vi "niRFUtil WFM Bit Correlator.vi"(3 "Samples (-1 = All)":i32=-1, 4 "Bit Mask":T1 min=0, 5 "Bit Stream In":T1 min=0) -> (1 "Sync Index":u32, 2 "Bit Stream Out":T1 min=0)   [LabVIEW 2015, in "niRFUtil.lvlib"]
doc: "(c) Copyright 2006, National Instruments, Inc. This VI may not be duplicated, sold, or distributed without written consent from National Instruments."
uses:
  niRFUtil.lvlib
  Includes/niRFUtil INC Bit Array.ctl
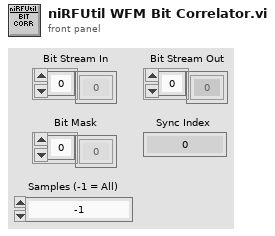
[diagram p1: front panel]
types:
  T1 = typedef "niRFUtil.lvlib/niRFUtil INC Bit Array.ctl" = i8[]
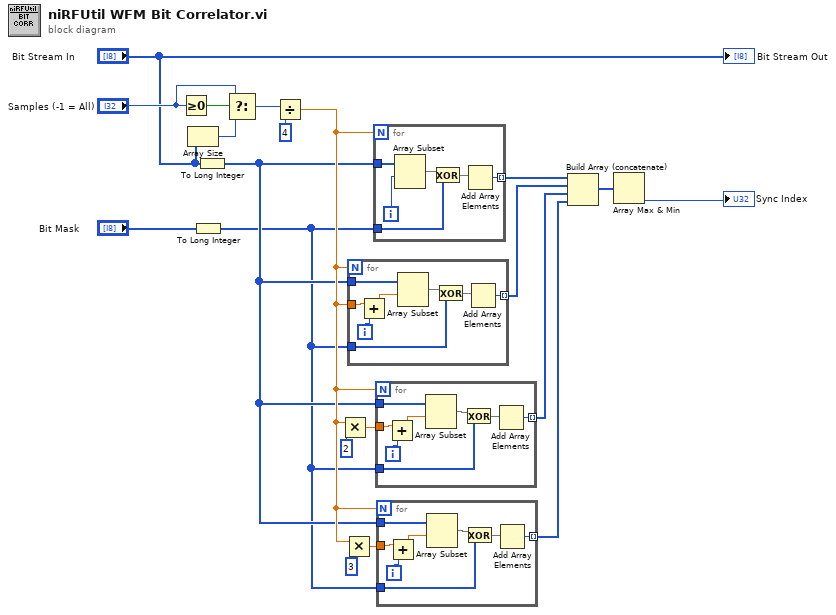
[diagram p0: block diagram]
diagram:
  n1 = Greater Or Equal To 0?(x="Samples (-1 = All)") -> (x >= 0?=w10:bool)
  n2 = Array Size(array="Bit Stream In") -> (size(s)=w9:i32)
  n3 = To Long Integer(number="Bit Mask") -> (32bit integer=w1:i32[])
  n4 = To Long Integer(number="Bit Stream In") -> (32bit integer=w2:i32[])
  n5 = Select(t="Samples (-1 = All)", s=w10, f=w9) -> (s? t:f=w8:i32)
  n6 = Divide(x=w8, y=4 ("x")) -> (x/y=w12:dbl)
  n7 = Multiply(x=w12, y=2) -> (x*y=w18:dbl)
  n8 = Multiply(x=w12, y=3) -> (x*y=w16:dbl)
  n9 = for {
    N: w12 -> [_]
    tunnel: w2 -> [w26]
    tunnel: w1 -> [w23]
    tunnel: [w27] -> w19 mode=indexing
    tunnel: w12 -> [w21]
    i -> [w24]
    n10 = Add(x=w21, y=w24) -> (x+y=w22:dbl)
    n11 = Array Subset(array=w26, index=w22) -> (w25:i32[])  [unwired: 1 in]
    n12 = Exclusive Or(1:w23, 2:w25) -> (0:w28:i32[])
    n13 = Add Array Elements(numeric array=w28) -> (sum=w27:i32)
  }
  n14 = for {
    N: w12 -> [_]
    tunnel: w2 -> [w32]
    tunnel: w1 -> [w29]
    tunnel: [w33] -> w20 mode=indexing
    i -> [w30]
    n15 = Array Subset(array=w32, index=w30) -> (w31:i32[])  [unwired: 1 in]
    n16 = Exclusive Or(1:w29, 2:w31) -> (0:w34:i32[])
    n17 = Add Array Elements(numeric array=w34) -> (sum=w33:i32)
  }
  n18 = for {
    N: w12 -> [_]
    tunnel: w2 -> [w40]
    tunnel: w1 -> [w37]
    tunnel: [w41] -> w14 mode=indexing
    tunnel: w18 -> [w35]
    i -> [w38]
    n19 = Add(x=w35, y=w38) -> (x+y=w36:dbl)
    n20 = Array Subset(array=w40, index=w36) -> (w39:i32[])  [unwired: 1 in]
    n21 = Exclusive Or(1:w37, 2:w39) -> (0:w42:i32[])
    n22 = Add Array Elements(numeric array=w42) -> (sum=w41:i32)
  }
  n23 = for {
    N: w12 -> [_]
    tunnel: w2 -> [w48]
    tunnel: w1 -> [w45]
    tunnel: [w49] -> w13 mode=indexing
    tunnel: w16 -> [w43]
    i -> [w46]
    n24 = Add(x=w43, y=w46) -> (x+y=w44:dbl)
    n25 = Array Subset(array=w48, index=w44) -> (w47:i32[])  [unwired: 1 in]
    n26 = Exclusive Or(1:w45, 2:w47) -> (0:w50:i32[])
    n27 = Add Array Elements(numeric array=w50) -> (sum=w49:i32)
  }
  n28 = Build Array (concatenate)(w20, w19, w14, w13) -> (w4:i32[])
  n29 = Array Max & Min(array=w4) -> (min index (indices)=→"Sync Index":i32)  [unwired: 3 out]
  "Bit Stream Out" <- "Bit Stream In"
